vi "Parse UDP String (Vision).vi"(1 "UDP Packet In":string) -> (0 "Array":dbl[][](array[numeric]))   [LabVIEW 2011]
panel:
  out "error out":errorcluster
  in  "Regex":string="\\d+\\.\\d+"
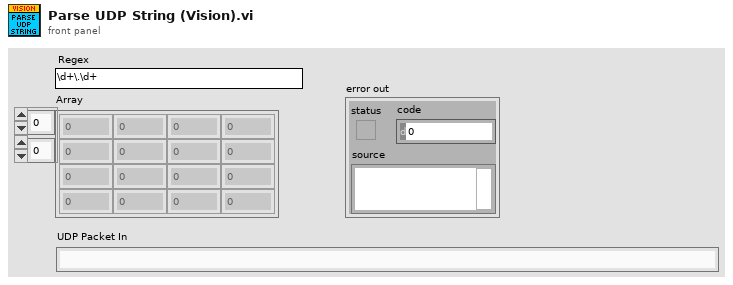
[diagram p1: front panel]
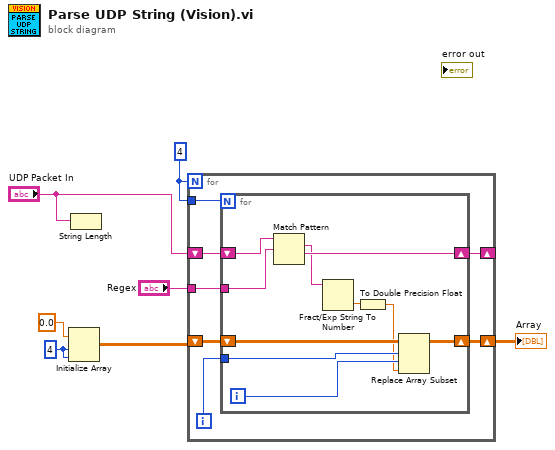
[diagram p0: block diagram]
diagram:
  w4 = 4
  w7 = 4 ("dimension size")
  n1 = Initialize Array(0.0, w7, w7) -> (w5:dbl[][])
  n2 = String Length(string="UDP Packet In") -> ()  [unwired: 1 out]
  n3 = for {
    N: w4 -> [_]
    shift-right: [w13] -> _
    shift-left: "UDP Packet In" -> [w14]
    tunnel: "Regex" -> [w12]
    tunnel: w4 -> [w9]
    shift-right: [w8] -> w3
    shift-left: w5 -> [w11]
    i -> [w10]
    n4 = for {
      N: w9 -> [_]
      shift-right: [w24] -> w13
      shift-left: w14 -> [w23]
      tunnel: w12 -> [w22]
      tunnel: w10 -> [w18]
      shift-right: [w15] -> w8
      shift-left: w11 -> [w19]
      i -> [w17]
      n5 = Match Pattern(string=w23, regular expression=w22) -> (match substring=w21:string, after substring=w24:string)  [unwired: 1 in, 2 out]
      n6 = Fract/Exp String To Number(string=w21) -> (number=w20:dbl)  [unwired: 3 in, 1 out]
      n7 = To Double Precision Float(number=w20) -> (double precision float=w16:dbl)
      n8 = Replace Array Subset(array=w19, new element=w16, index (row)=w18, index (col)=w17) -> (w15:dbl[][])
    }
  }
  "Array" <- w3
